vi "Initialize.vi"(7 "Serial Configuration":T1={"Baud Rate"=9600, "Parity"=0, "Data Bits"=8, "Stop Bits"=10, "Flow Control"=0} {"Flow Control" items=["None", "XON/XOFF", "RTS/CTS", "XON/XOFF & RTS/CTS", "DTR/DSR", "XON/XOFF & DTR/DSR"]; "Stop Bits" items=["1.0"=10, "1.5"=15, "2.0"=20]; "Data Bits" items=["7"=7, "8"=8]; "Parity" items=["None", "Odd", "Even", "Mark", "Space"]; "Baud Rate" items=["300"=300, "600"=600, "1200"=1200, "2400"=2400, "4800"=4800, "9600"=9600, "19200"=19200]}, 8 "error in (no error)":errorcluster, 9 "Reset (True)":bool=TRUE, 10 "ID Query (True)":bool=TRUE, 11 "VISA resource name":refnum<visa-resource-name>) -> (0 "error out":errorcluster, 3 "VISA resource name out":refnum<visa-resource-name>)   [LabVIEW 2015, in "Fluke 8808.lvlib"]
doc: "Establishes communication with the instrument and optionally performs an instrument identification query and/or an instrument reset. It also places the instrument in a default state needed for other instrument driver operations. Therefore, call this VI before calling other instrument driver VIs for this instrument. Generally, you need to call the Initialize VI only once at the beginning of an application."
uses:
  <instrlib>/Fluke 8808/Fluke 8808.lvlib
panel:
  # "(c) 2009 National Instruments.  ALL RIGHTS RESERVED."
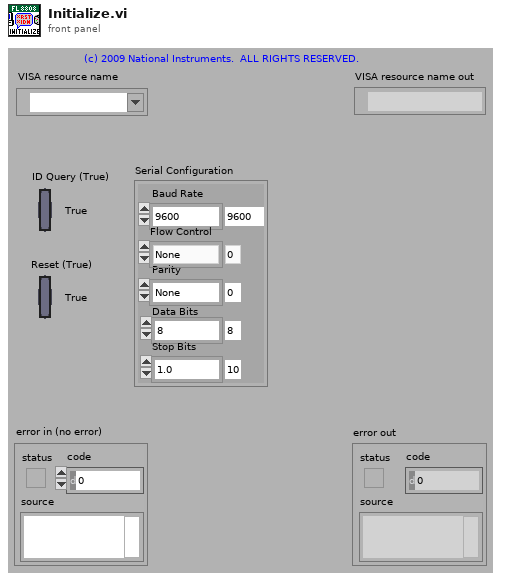
[diagram p1: front panel]
types:
  T1 = cluster{"Baud Rate":u32, "Parity":u16, "Data Bits":u16, "Stop Bits":u16, "Flow Control":u16}
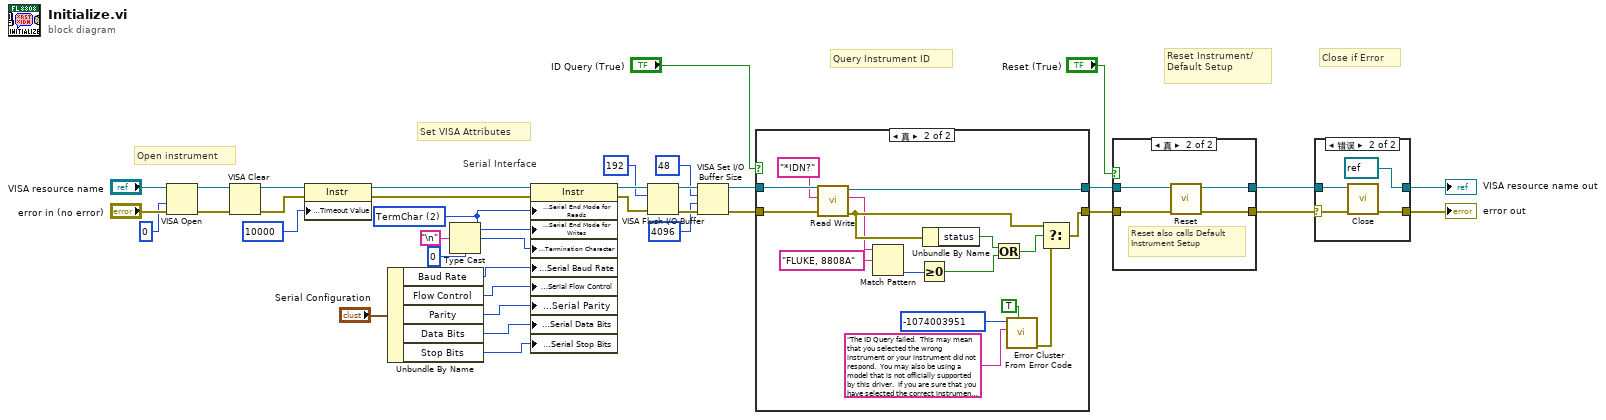
[diagram p0: block diagram]
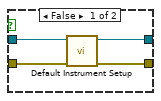
[diagram p3: hidden frame]
diagram:
  w10 = u16 2 items=["None", "LastBit", "TermChar"] ("Serial Settings:Serial End Mode for Reads")
  # "Serial Interface"
  # "Set VISA Attributes"
  # "Close if Error"
  # "Query Instrument ID"
  # "Reset Instrument/\nDefault Setup"
  # "Open instrument"
  n1 = VISA Open(access mode=u32 0, error in (no error)="error in (no error)", VISA resource name="VISA resource name") -> (VISA resource name=w25:refnum<visa-resource-name>, error out=w24:errorcluster)  [unwired: 2 in]
  n2 = VISA Clear(VISA resource name=w25, error in (no error)=w24) -> (VISA resource name out=w23:refnum<visa-resource-name>, error out=w22:errorcluster)
  n3 = property class="Instr"(reference=w23, error in=w22, "General Settings:Timeout Value"=u32 10000) -> (reference out=w28:refnum<visa-resource-name>, error out=w27:errorcluster)
  n4 = Unbundle By Name("Serial Configuration") -> ("Baud Rate"=w8:u32, "Flow Control"=w4:u16, "Parity"=w6:u16, "Data Bits"=w7:u16, "Stop Bits"=w3:u16)
  n5 = Type Cast(type=u8 0, x="\n" ("Line Feed Constant")) -> (*(type *) &x=w9:u8)
  n6 = property class="Instr"(reference=w28, error in=w27, "Serial Settings:Serial End Mode for Reads"=w10, "Serial Settings:Serial End Mode for Writes"=w10, "Message Based Settings:Termination Character"=w9, "Serial Settings:Serial Baud Rate"=w8, "Serial Settings:Serial Flow Control"=w4, "Serial Settings:Serial Parity"=w6, "Serial Settings:Serial Data Bits"=w7, "Serial Settings:Serial Stop Bits"=w3) -> (reference out=w16:refnum<visa-resource-name>, error out=w18:errorcluster)
  n7 = VISA Flush I/O Buffer(VISA resource name=w16, mask (16)=u16 192, error in (no error)=w18) -> (VISA resource name out=w19:refnum<visa-resource-name>, error out=w17:errorcluster)
  n8 = VISA Set I/O Buffer Size(VISA resource name=w19, mask (16)=u16 48, size (4096)=u32 4096 ("size (0)"), error in (no error)=w17) -> (VISA resource name out=w30:refnum<visa-resource-name>, error out=w29:errorcluster)
  n9 = case shown="真" "ID Query (True)" {
    tunnel: [w38 w55] -> w36
    tunnel: [w39 w42] -> w37
    tunnel: w30 -> [w39 w45]
    tunnel: w29 -> [w38 w44]
    frame False {
    }
    frame True {
      n10 = call <instrlib>:"Read Write.vi"("error in (no error)"=w44, "Write String"="*IDN?", "VISA resource name"=w45) -> ("error out"=w43:errorcluster, "Read Data"=w41:string, "VISA resource name out"=w42:refnum<visa-resource-name>)  [unwired: 6 in]
      n11 = Match Pattern(string=w41, regular expression="FLUKE, 8808A") -> (offset past match=w49:i32)  [unwired: 1 in, 3 out]
      n12 = Greater Or Equal To 0?(x=w49) -> (x >= 0?=w47:bool)
      n13 = Unbundle By Name(w43) -> ("status"=w48:bool)
      n14 = Or(x=w48, y=w47) -> (x .or. y?=w46:bool)
      n15 = call <vilib>:"Error Cluster From Error Code.vi"("show call chain? (False)"=TRUE, "error message (\"\")"="The ID Query failed.  This may mean that you selected the wrong instrument or your instrument did not respond.  You may also be using a model that is not officially supported by this driver.  If you are sure that you have selected the correct instrument and it is responding, try disabling the ID Query." ("Source (VI Name)"), "error code (0)"=-1074003951 ("Code")) -> ("error out"=w53:errorcluster)  [unwired: 6 in]
      n16 = Select(t=w43, s=w46, f=w53) -> (s? t:f=w55:errorcluster)
    }
  }
  n17 = case shown="真" "Reset (True)" {
    tunnel: w36 -> [w58 w60]
    tunnel: [w56 w63] -> w1
    tunnel: w37 -> [w59 w61]
    tunnel: [w57 w62] -> w2
    frame False {
      n18 = call <instrlib>:"Default Instrument Setup.vi"("error in (no error)"=w58, "VISA resource name"=w59) -> ("error out"=w56:errorcluster, "VISA resource name out"=w57:refnum<visa-resource-name>)  [unwired: 8 in]
    }
    frame True {
      # "Reset also calls Default Instrument Setup"
      n19 = call <instrlib>:"Reset.vi"("error in (no error)"=w60, "VISA resource name"=w61) -> ("error out"=w63:errorcluster, "VISA resource name out"=w62:refnum<visa-resource-name>)  [unwired: 8 in]
    }
  }
  n20 = case shown="错误" w1 {
    selector: w1 -> [w64 w67]
    tunnel: w2 -> [w65 w68]
    tunnel: [w65 refnum<visa-resource-name> refnum ("VISA resource name out")] -> w21
    tunnel: [w64 w69] -> w20
    frame No Error {
    }
    frame Error {
      n21 = call <instrlib>:"Close.vi"("error in (no error)"=w67, "VISA resource name"=w68) -> ("error out"=w69:errorcluster)  [unwired: 9 in]
    }
  }
  "VISA resource name out" <- w21
  "error out" <- w20
